vi "ControlTerminal.vi"(8 "error in":errorcluster, 11 "reference":refnum<vi>) -> (0 "error out":errorcluster, 3 "ControlTerminal out":refnum<class "ControlTerminal.lvclass">)   [LabVIEW 2014, in "Raspberry Pi Compatible Compiler for LabVIEW.lvlib" / "ControlTerminal.lvclass"]
uses:
  ControlTerminal.lvclass
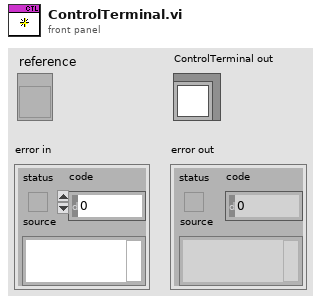
[diagram p1: front panel]
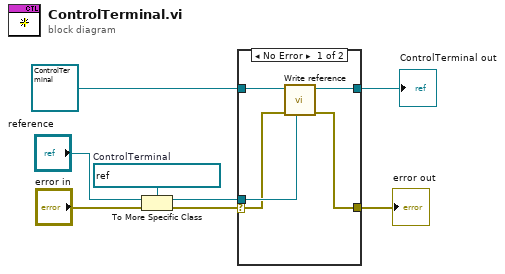
[diagram p0: block diagram]
diagram:
  w6 = refnum<vi> refnum  # ControlTerminal
  n1 = To More Specific Class(target class=w6, reference="reference", error in="error in") -> (specific class reference=w3:refnum<vi>, error out=w4:errorcluster)
  n2 = case shown="No Error" w4 {
    selector: w4 -> [w11 w14]
    tunnel: refnum<class "ControlTerminal.lvclass"> refnum ("ControlTerminal in") -> [w13 w15]
    tunnel: w3 -> [w12 _]
    tunnel: [w10 w15] -> w2
    tunnel: [w9 w14] -> w1
    frame No Error {
      n3 = call-dynamic "Write reference.vi"("reference"=w12, "error in"=w11, "GObject in"=w13) -> ("error out"=w9:errorcluster, "GObject out"=w10:refnum<class "ControlTerminal.lvclass">)  [unwired: 5 in]
    }
    frame Error {
    }
  }
  "error out" <- w1
  "ControlTerminal out" <- w2
